vi "Pre Launch Init.vi"(11 "Network Actor in":refnum<class "Network Actor.lvclass">) -> (0 "error out":errorcluster, 3 "Network Actor out":refnum<class "Network Actor.lvclass">)   [LabVIEW 2014, in "Network Actor Library.lvlib" / "Network Actor.lvclass"]
doc: "(<B>Filename</B>: Actor Framework.lvlib:Actor.lvclass:Pre Launch Init.vi)\n\nDefines behavior that occurs after the Launch Nested Actor method is invoked but before the actor's Actor Core method begins running.\n\nBy default, this method does nothing. A descendant class may override it to define behavior."
uses:
  Network Actor.lvclass
  reusable/Session APIs/File Access/Config Data/Config Data.lvclass
  <vilib>/Utility/config.llb/NI_LVConfig.lvlib
  <vilib>/Utility/config.llb/Read Key (String).vi
  <vilib>/Utility/config.llb/Read Key (U32).vi
  reusable/Session APIs/Session Log/System Log.lvclass
  <vilib>/Utility/config.llb/Read Key (Path).vi
  <vilib>/Utility/tcp.llb/UDP Multicast Read-Only Open.vi
  SuperActor/SuperActor.lvclass
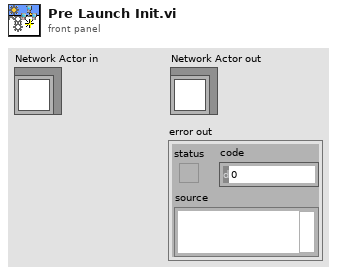
[diagram p1: front panel]
types:
  T1 = typedef "Session - Root.lvclass/Session Handle.ctl" = refnum<data-value>
  T2 = typedef "NI_LVConfig.lvlib/Config Data RefNum.ctl" = refnum<k1>
  T3 = cluster{"ID":string, "DataDescr":cluster{"Type":string, "Name":string, "Write":bool}[]}[]
  T4 = cluster{"Type":string, "Name":string, "Write":bool}[]
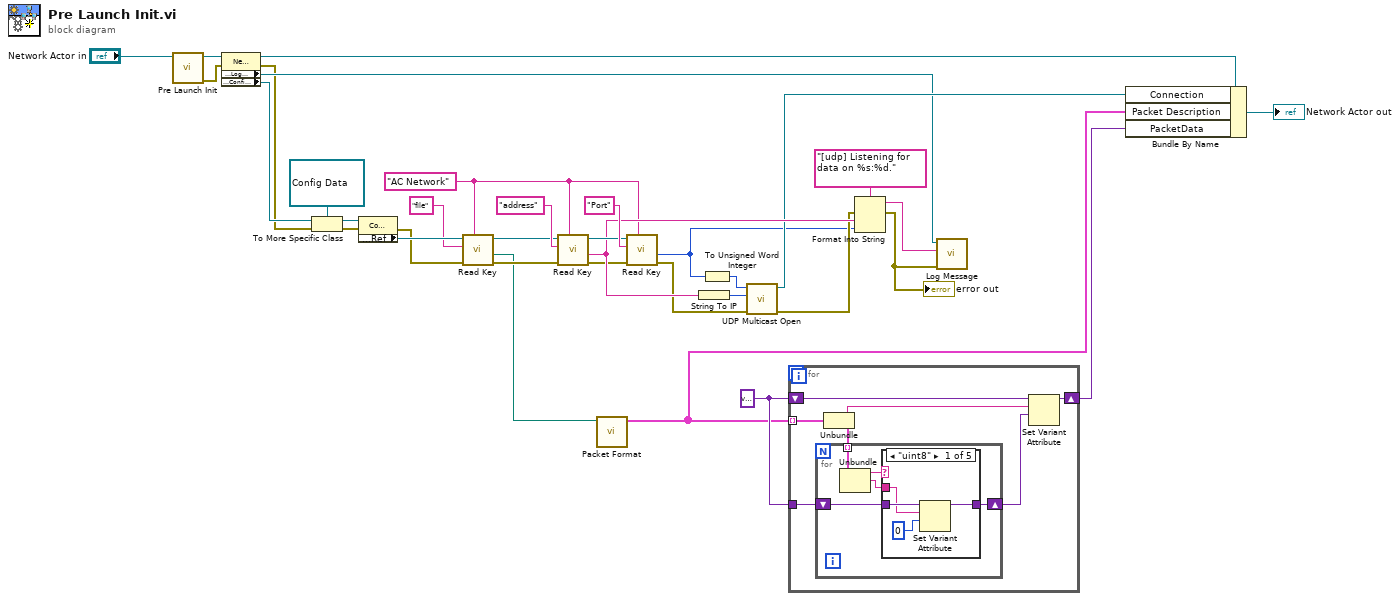
[diagram p0: block diagram]
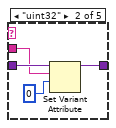
[diagram p2: hidden frame]
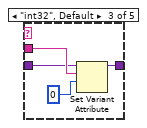
[diagram p3: hidden frame]
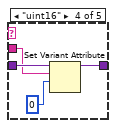
[diagram p4: hidden frame]
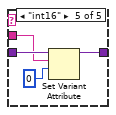
[diagram p5: hidden frame]
diagram:
  w12 = variant
  w17 = "AC Network" ("section")
  n1 = call-parent "Pre Launch Init.vi"("Ex Nested in"="Network Actor in") -> ("error out"=w2:errorcluster, "Ex Nested out"=w6:refnum<class "Network Actor.lvclass">)  [unwired: 9 in]
  n2 = property class="Network Actor"(reference=w6, error in=w2) -> (reference out=w3:refnum<class "Network Actor.lvclass">, error out=w1:errorcluster, "Accessors:Log Session"=w4:T1, "Accessors:Config Session"=w5:T1)
  n3 = To More Specific Class(target class=refnum<data-value> refnum ("Session Handle"), reference=w5, error in=w1) -> (specific class reference=w34:refnum<data-value>, error out=w33:errorcluster)
  n4 = property class="Config Data"(reference=w34, error in=w33) -> (error out=w14:errorcluster, "Accessors:Ref"=w19:T2)  [unwired: 1 out]
  n5 = call-poly <vilib>:"Read Key.vi"("section"=w17, "error in (no error)"=w14, "key"="file", "refnum"=w19) -> ("error out"=w15:errorcluster, "value"=w13:path, "refnum out"=w18:T2)  [unwired: 4 in, 1 out]
  n6 = call-poly <vilib>:"Read Key.vi"("section"=w17, "error in (no error)"=w15, "key"="address", "refnum"=w18) -> ("error out"=w24:errorcluster, "value"=w26:string, "refnum out"=w30:T2)  [unwired: 4 in, 1 out]
  n7 = call "Packet Format.vi"("value"=w13) -> ("data"=w10:T3)  [unwired: 9 in, 1 out]
  n8 = call-poly <vilib>:"Read Key.vi"("section"=w17, "error in (no error)"=w24, "key"="Port", "refnum"=w30) -> ("error out"=w23:errorcluster, "value"=w9:u32)  [unwired: 4 in, 2 out]
  n9 = String To IP(1:w26) -> (0:w29:u32)
  n10 = To Unsigned Word Integer(number=w9) -> (unsigned 16bit integer=w8:u16)
  n11 = call-poly <vilib>:"UDP Multicast Open.vi"("error in (no error)"=w23, "multicast addr"=w29, "port"=w8) -> ("error out"=w21:errorcluster, "connection ID"=w20:refnum<k16>)  [unwired: 6 in, 1 out]
  n12 = for {
    tunnel: w10 -> [w41] mode=indexing
    tunnel: w12 -> [w42]
    shift-right: [w36] -> w11
    shift-left: w12 -> [w39]
    n13 = Unbundle(w41) -> ("ID"=w40:string, "DataDescr"=w38:T4)
    n14 = for {
      tunnel: w38 -> [w47] mode=indexing
      shift-right: [w43] -> w37
      shift-left: w42 -> [w44]
      n15 = Unbundle(w47) -> ("Type"=w46:string, "Name"=w45:string)  [unwired: 1 out]
      n16 = case shown="\"uint8\"" w46 {
        tunnel: w45 -> [w48 w52 w59 w60 w64]
        tunnel: w44 -> [w50 w54 w58 w62 w66]
        tunnel: [w49 w53 w57 w61 w65] -> w43
        frame "uint8" {
          n17 = Set Variant Attribute(Variant=w50, name=w48, value=u8 0) -> (Variant out=w49:variant)  [unwired: 1 in, 2 out]
        }
        frame "uint32" {
          n18 = Set Variant Attribute(Variant=w54, name=w52, value=u32 0) -> (Variant out=w53:variant)  [unwired: 1 in, 2 out]
        }
        frame "int32", Default {
          n19 = Set Variant Attribute(Variant=w58, name=w59, value=0) -> (Variant out=w57:variant)  [unwired: 1 in, 2 out]
        }
        frame "uint16" {
          n20 = Set Variant Attribute(Variant=w62, name=w60, value=u16 0) -> (Variant out=w61:variant)  [unwired: 1 in, 2 out]
        }
        frame "int16" {
          n21 = Set Variant Attribute(Variant=w66, name=w64, value=i16 0) -> (Variant out=w65:variant)  [unwired: 1 in, 2 out]
        }
      }
    }
    n22 = Set Variant Attribute(Variant=w39, name=w40, value=w37) -> (Variant out=w36:variant)  [unwired: 1 in, 2 out]
  }
  n23 = Format Into String(format string="[udp] Listening for data on %s:%d.", error in=w21, w26, w9) -> (resulting string=w25:string, error out=w22:errorcluster)  [unwired: 1 in]
  "error out" <- w22
  n24 = call "Log Message.vi"("error in"=w22, "MSG In"=w25, "session in"=w4) -> ()  [unwired: 7 in, 2 out]
  n25 = Bundle By Name(cluster=w3, "Connection"=w20, "Packet Description"=w10, "PacketData"=w11) -> (→"Network Actor out":refnum<class "Network Actor.lvclass">)
